vi "sabertooth packetized [-1.1] speed to command, data.vi"(2 "Motor speed":dbl(knob) scale=-1.0..1.0, 3 "Motor to control":u8(ring) items=["Motor 1"=0, "Motor 2"=4]) -> (0 "data":u8, 1 "command":u8)   [LabVIEW 2018]
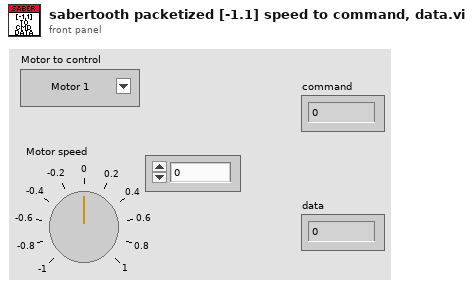
[diagram p1: front panel]
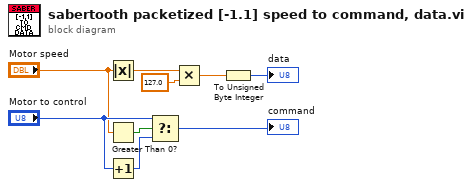
[diagram p0: block diagram]
diagram:
  n1 = Absolute Value(x="Motor speed") -> (abs(x)=w8:dbl)
  n2 = Greater Than 0?(x="Motor speed") -> (x > 0?=w6:bool)
  n3 = Increment(x="Motor to control") -> (x+1=w3:u8)
  n4 = Select(t="Motor to control", s=w6, f=w3) -> (s? t:f=→"command":u8)
  n5 = Multiply(x=w8, y=127.0) -> (x*y=w9:dbl)
  n6 = To Unsigned Byte Integer(number=w9) -> (unsigned 8bit integer=→"data":u8)
